vi "SI656_Generator_Power.vi"(0 "SI656 in":refnum<class "SI656.lvclass">, 2 "From Turbine":T2, 5 "error in (no error)":errorcluster) -> (14 "SI656 out":refnum<class "SI656.lvclass">, 16 "PG Factor":dbl, 17 "PG 2nd Min in %":dbl, 19 "error out":errorcluster)   [LabVIEW 2022 SP3, in "SI656.lvclass"]
uses:
  SI656.lvclass
  SI656.lvclass/SI656.ctl
panel:
  in  "Set Params 4":T1
  in  "Set Params 3":T1
  in  "Set Params 2":T1
  in  "Set Params":T1
  # "SI656"
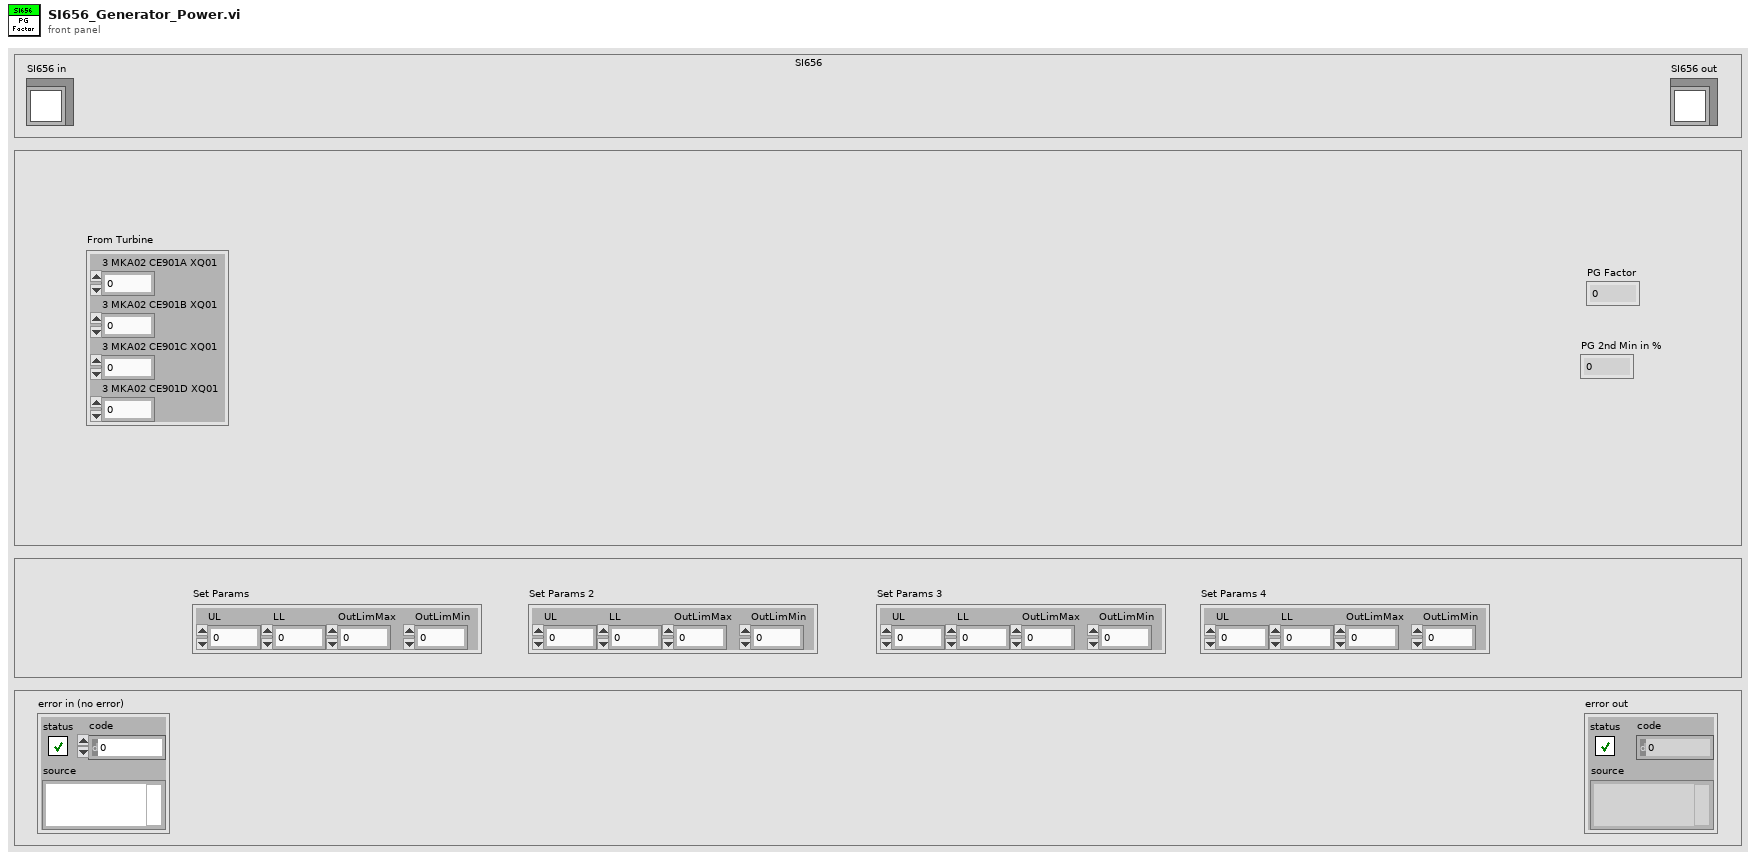
[diagram p1: front panel]
types:
  T1 = cluster{"UL":dbl, "LL":dbl, "OutLimMax":dbl, "OutLimMin":dbl}
  T2 = cluster{"3 MKA02 CE901A XQ01":dbl, "3 MKA02 CE901B XQ01":dbl, "3 MKA02 CE901C XQ01":dbl, "3 MKA02 CE901D XQ01":dbl}
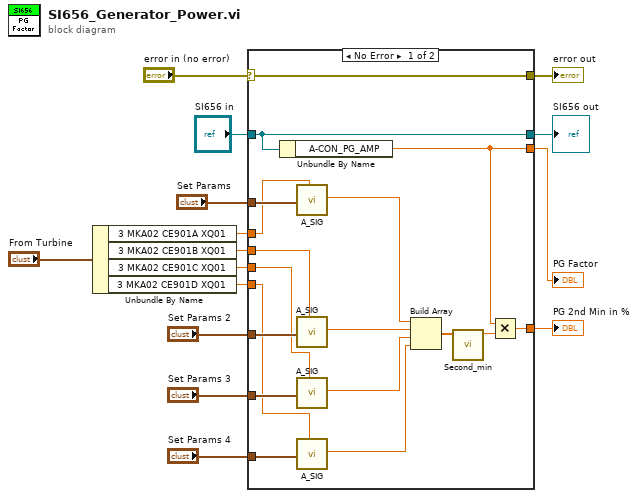
[diagram p0: block diagram]
diagram:
  n1 = Unbundle By Name("From Turbine") -> ("3 MKA02 CE901A XQ01"=w8:dbl, "3 MKA02 CE901B XQ01"=w7:dbl, "3 MKA02 CE901C XQ01"=w6:dbl, "3 MKA02 CE901D XQ01"=w5:dbl)
  n2 = case shown="No Error" "error in (no error)" {
    selector: "error in (no error)" -> [w33 w35]
    tunnel: [w33 w35] -> w14
    tunnel: [w32 w34] -> w12
    tunnel: "SI656 in" -> [w32 w34]
    tunnel: [w26 _] -> w11
    tunnel: w5 -> [w16 _]
    tunnel: w6 -> [w17 _]
    tunnel: w7 -> [w18 _]
    tunnel: w8 -> [w19 _]
    tunnel: [w24 _] -> w10
    tunnel: "Set Params" -> [w23 _]
    tunnel: "Set Params 2" -> [w22 _]
    tunnel: "Set Params 3" -> [w21 _]
    tunnel: "Set Params 4" -> [w20 _]
    frame No Error {
      n3 = Unbundle By Name(w32) -> ("A-CON_PG_AMP"=w26:dbl)
      n4 = call "A_SIG.vi"("Set Params"=w23, "Input"=w19) -> ("A_SIG_out"=w31:dbl)  [unwired: 16 in, 1 out]
      n5 = call "A_SIG.vi"("Set Params"=w22, "Input"=w18) -> ("A_SIG_out"=w30:dbl)  [unwired: 16 in, 1 out]
      n6 = call "A_SIG.vi"("Set Params"=w21, "Input"=w17) -> ("A_SIG_out"=w29:dbl)  [unwired: 16 in, 1 out]
      n7 = call "A_SIG.vi"("Set Params"=w20, "Input"=w16) -> ("A_SIG_out"=w28:dbl)  [unwired: 16 in, 1 out]
      n8 = Build Array(w31, w30, w29, w28) -> (w27:dbl[])
      n9 = call "Second_min.vi"("Array"=w27) -> ("output"=w25:dbl)  [unwired: 9 in, 1 out]
      n10 = Multiply(x=w26, y=w25) -> (x*y=w24:dbl)
    }
    frame Error {
    }
  }
  "error out" <- w14
  "SI656 out" <- w12
  "PG Factor" <- w11
  "PG 2nd Min in %" <- w10
